vi "OriginSearch.vi"(5 "HomeMode":string[](array[string])=["4", "4", "0"], 7 "#Axis":i32, 8 "error in":errorcluster, 11 "VISA resource":refnum<visa-resource-name>) -> (0 "error out":errorcluster)   [LabVIEW 2012, in "ESP300.lvlib"]
uses:
  <instrlib>/ESP300/ESP300.lvlib
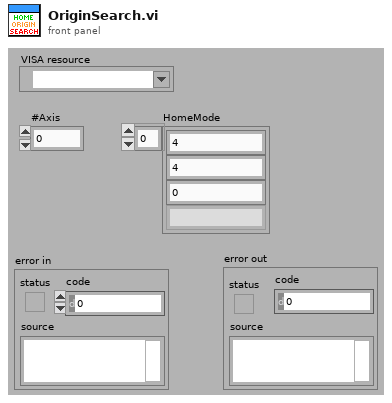
[diagram p1: front panel]
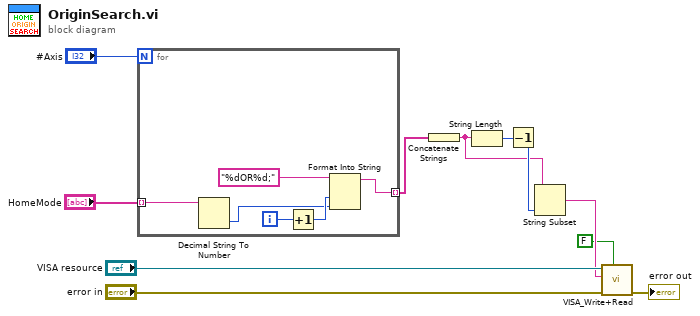
[diagram p0: block diagram]
diagram:
  n1 = for {
    N: "#Axis" -> [_]
    tunnel: [w17] -> w3 mode=indexing
    tunnel: "HomeMode" -> [w13] mode=indexing
    i -> [w16]
    n2 = Decimal String To Number(string=w13) -> (number=w12:i32)  [unwired: 2 in, 1 out]
    n3 = Increment(x=w16) -> (x+1=w15:i32)
    n4 = Format Into String(format string="%dOR%d;", w15, w12) -> (resulting string=w17:string)  [unwired: 2 in, 1 out]
  }
  n5 = Concatenate Strings(w3) -> (w4:string)
  n6 = String Length(string=w4) -> (length=w6:i32)
  n7 = Decrement(x=w6) -> (x-1=w5:i32)
  n8 = String Subset(string=w4, length (rest)=w5) -> (substring=w7:string)  [unwired: 1 in]
  n9 = call <instrlib>:"VISA_Write+Read.vi"("Read?(T)"=FALSE ("Read?"), "error in (no error)"="error in", "Write Buffer"=w7, "VISA resource name"="VISA resource") -> ("error out"=→"error out":errorcluster)  [unwired: 5 in, 2 out]
